vi "ReadFound.vi"(8 "error in (no error)":errorcluster, 11 "object in":refnum<class "inspect_reply Message.lvclass">) -> (0 "error out":errorcluster, 2 "found":bool, 3 "object out":refnum<class "inspect_reply Message.lvclass">)   [LabVIEW 2018, in "ClientMessaging.lvlib" / "inspect_reply Message.lvclass"]
uses:
  inspect_reply Message.lvclass
  inspect_reply Message.lvclass/inspect_reply Message.ctl
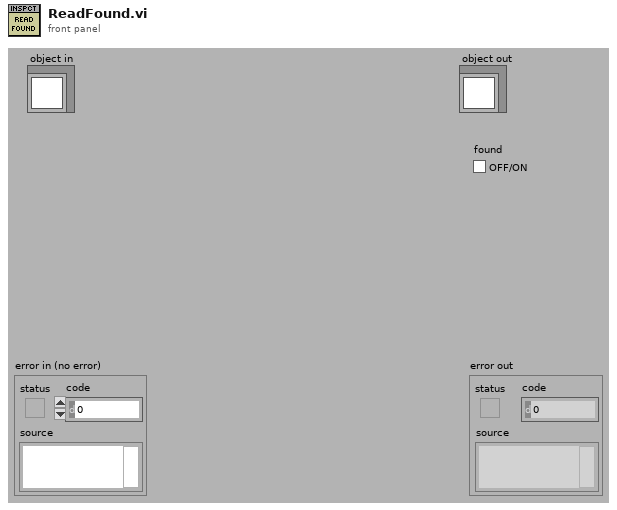
[diagram p1: front panel]
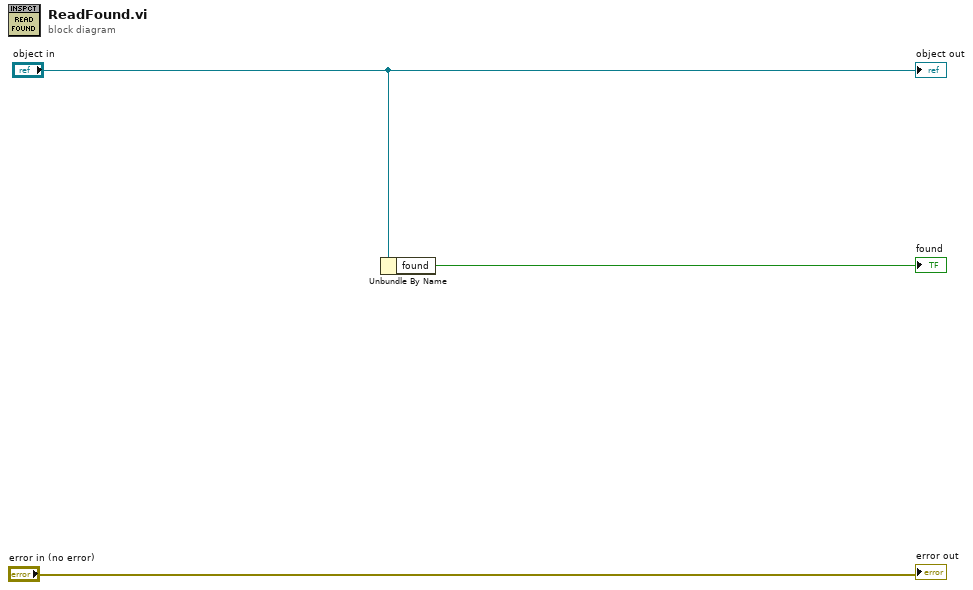
[diagram p0: block diagram]
diagram:
  n1 = Unbundle By Name("object in") -> ("found"=→"found":bool)
  "error out" <- "error in (no error)"
  "object out" <- "object in"
